vi "Average_flow_x_time.vi"(9 "Array of timestamps":timestamp[](array[timestamp]), 10 "Previous Flow":dbl, 11 "Latest Flow":dbl) -> (3 "Volume (SL)":dbl)   [LabVIEW 2018]
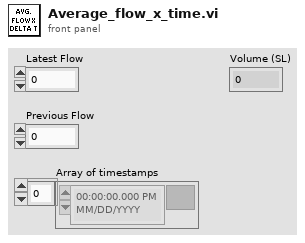
[diagram p1: front panel]
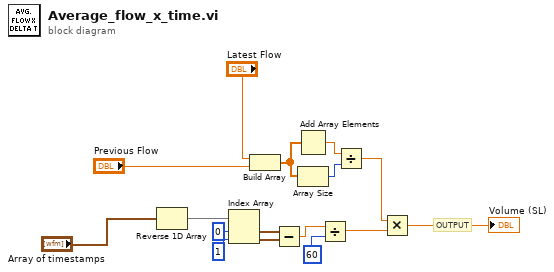
[diagram p0: block diagram]
diagram:
  # "OUTPUT"
  n1 = Reverse 1D Array(array="Array of timestamps") -> (reversed array=w4:timestamp[])
  n2 = Index Array(array=w4, index #1=0 ("index"), index #2=1 ("index")) -> (element #1=w7:timestamp, element #2=w8:timestamp)
  n3 = Build Array("Latest Flow", "Previous Flow") -> (w13:dbl[])
  n4 = Subtract(x=w7, y=w8) -> (x-y=w10:dbl)
  n5 = Add Array Elements(numeric array=w13) -> (sum=w12:dbl)
  n6 = Array Size(array=w13) -> (size(s)=w11:i32)
  n7 = Divide(x=w10, y=60) -> (x/y=w2:dbl)
  n8 = Divide(x=w12, y=w11) -> (x/y=w16:dbl)
  n9 = Multiply(x=w16, y=w2) -> (x*y=→"Volume (SL)":dbl)
